vi "AlliGator Save All Decay Fit Parameter Maps to ASCII.vi"(8 "error in (no error)":errorcluster, 11 "Data Value Reference in":refnum<data-value>) -> (0 "error out":errorcluster, 3 "Data Value Reference out":refnum<data-value>)   [LabVIEW 2021, in "AlliGator Decay Fit Parameter Map.lvlib"]
doc: "Saves the Decay Fir Parameter Map 2D array to an ASCII file."
uses:
  AlliGator Decay Fit Parameter Map.lvlib
  AlliGator Internal Variables v2.ctl
  <vilib>/vision/Image Controls.llb/IMAQ Image.ctl
  AlliGator Gate Image Set.ctl
  AlliGator FLI Dataset Type.ctl
  AlliGator Data Series Type.ctl
  AlliGator Dataset Channel.ctl
  AlliGator Gate Arithmetic.ctl
  AlliGator Displayed Image.ctl
  Image/Named ROI Description.ctl
  AlliGator Decay Metadata v3.ctl
  AlliGator Decay Background Subtraction Info.ctl
  AlliGator Baseline Subtraction Method.ctl
  Graphs/XY Graph/XY Graph Plot Shift Parameters.ctl
  Graphs/XY Graph/XY Graph Plot Shift Method.ctl
  AlliGator Decay Extrapolation Parameters.ctl
  Phasor/Calibration Phasor (m, phi).ctl
  Phasor/Phasor Reference Series.ctl
  Phasor/Phasor Calibration Map v2.ctl
  Phasor/Phasor (g, s).ctl
  AlliGator Raw Phasor Plot Data v4.ctl
  Phasor/Phasor Standard Deviation Options.ctl
  AlliGator Phasor Multi-Harmonic Data.ctl
  Phasor/Phasor Harmonic Data.ctl
  AlliGator Decay Fit Options & Parameters v2.ctl
  Fits/IRF(X)PSED/Decay Fit Options v2.ctl
  Fits/Decay Convolution/Decay Model.ctl
  Fits/Residual Type.ctl
  Fits/IRF(X)PSED/Fit Weights Type.ctl
  Fits/Non-linear Fitting Method v2.ctl
  Fits/Fit Calculation Method.ctl
  Fits/Non-linear Fitting Algorithm.ctl
  AlliGator Decay Fit Parameter Constraints 2.ctl
  Fits/IRF(X)PSED/Decay Fit Parameters In List.ctl
  Fits/IRF(X)PSED/MLE Baseline Offset Type.ctl
  AlliGator Decay Preprocessing Parameters.ctl
  Fits/IRF(X)PSED/Decay Fit Parameters & Derived Quantities List.ctl
  AlliGator Parameter Maps Data.ctl
  AlliGator Variables List.ctl
  Variant/Variant to Data/Variant to U16.vi
  <vilib>/Utility/file.llb/Write Delimited Spreadsheet (DBL).vi
  AlliGator Files.lvlib
  Files/Files.lvlib
  Strings/Strings.lvlib
  GUI/GUI.lvlib
  Error/Error.lvlib
  Notebook/Notebook.lvlib
  Rich Text Box/Rich Text Box.lvlib
  AlliGator Globals, Variables & Constants.lvlib
  Variant/Variant to Data/Variant to Data.lvlib
  Phasor/Phasor.lvlib
  Image/Image.lvlib
  AlliGator Decay Preprocessing.lvlib
  Graphs/XY Graph/XY Graph Add-Ons.lvlib
  AlliGator Phasor Graph.lvlib
  AlliGator Phasor Plot.lvlib
  AlliGator Source Image.lvlib
  Fits/Fits.lvlib
  AlliGator Internal Variables.lvlib
  AlliGator Decay Fit.lvlib
  AlliGator Settings.lvlib
  AlliGator Dual-Channel Datasets.lvlib
panel:
  # "see the AlliGator License on the block diagram (Ctrl+E or Window:Show Block Diagram)"
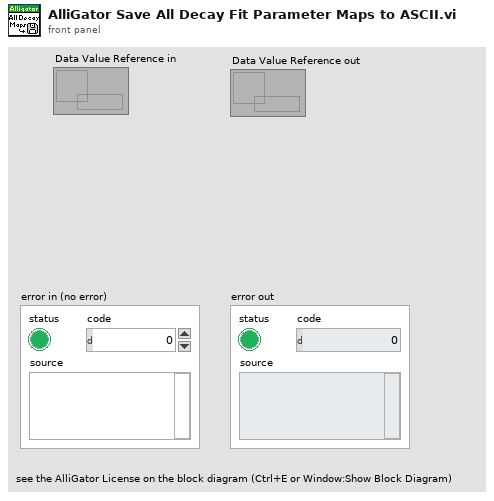
[diagram p1: front panel]
types:
  T1 = typedef "AlliGator Globals, Variables & Constants.lvlib/AlliGator Variables List.ctl" = enum16{"---- GUI ----", "GUI:Initialization Status", "GUI:State Indicators Refnum", "GUI:Original AlliGator Menu Items", "GUI:Current Action Loop State", "GUI:Script in progress", "GUI:Playback", "GUI:Loop Playback", "GUI:Search ROI Used", "GUI:Search ROI", "Decay Graph Max Legend Size", "Intensity Graph Max Legend Size", "Decay Statistics Graph Max Legend Size", "Phasor Graph Max Legend Size", "Phasor Ratio Graph Max Legend Size", "Lifetime Graph Max Legend Size", "---- Files ----", "Files:Export Dataset Frames as Individual Files", "Files:Show Batch Export Help Balloons", "Files:Frames in Dataset", "Files:ptu File Frame Start Indices", "Files:Current Frame in Dataset", "Files:Current Frame Timestamp", "Files:Dataset Loaded", "Files:Dataset Metadata", "Files:Dataset Channel", "Files:Dataset Data Description", "Files:Background Dataset Metadata", "Files:Background Dataset Channel", "Files:Background Dataset Data Description", "Files:Background File Subtraction", "Files:Background File Path", "Files:Background File Pile-up Correction", "Files:Background File Pixel Well Capacity", "Files:Background File Scaling Factor", "Files:Current Dataset Load Settings", "Files:Dataset Path", "Files:ICCD-specific Information", "Files:Macrotime Gate Separation", "------ Python Plugins ------", "Python Plugins:Information", "Python Plugins:Python Session", "Python Plugins:Valid Python Session?", "---- Source Image ----", "Source Image:ROIs", "Source Image:Current ROI", "Source Image:ROI Event Refnum", "X_Source Image Display Range", "X_Source Image Palette Information", "X_Type of Displayed Image", "X_Time Gate Slider", "Source Image:Palette List", "Source Image:Scale", "Source Image:ROI Overlay Color", "Source Image:Overlay to Erase", "Source Image:Is Displayed Image Accumulated", "Source Image:White Light Image Modified", "Source Image:Mask Image Modified", "---- Image Profile Window ----", "Image Profile:Window Event Refnum", "Image Profile:IntensityType", "Image Profile:Intensity Average Type", "Image Profile:Intensity-weighted SDV", "Image Profile:Box Profile Type", "Image Profile:Window Open", "Image Profile:Plotted Fit Parameter", "------ Phasor Graph -------", "Phasor Graph:Show Line", "---- Phasor Plot ---", "Phasor Plot:Parameters Changed", "Phasor Plot:FLI Dataset Modified since last Calculation", "Phasor Harmonics Data", "Selected Phasor Harmonics", "Phasor Harmonic Manager Event Refnum", "Phasor Plot:ROIs", "Phasor Plot:Current ROI", "Phasor Plot:ROI Event Refnum", "Phasor Plot:Image Reference Points", "Phasor Plot:Computed", "Phasor Plot:Palette Information", "Phasor Plot:Palette List", "Phasor Plot:Phasor Ratio Palette Information", "Phasor Plot:Phasor Ratio Palette List", "Phasor Plot:Image Scale", "Phasor Plot:Image Overlay to Erase", "Phasor Plot:Image Elements to Update", "Phasor Plot:Current Calculation Parameters", "Phasor Plot:Current Calibration Options", "Phasor Plot:Reset Cumulated Phasor Plot", "Phasor Plot:Reference 1", "Phasor Plot:Lifetime Reference 1", "Phasor Plot:Reference 1 Frequency", "Phasor Plot:Reference 2", "Phasor Plot:Lifetime Reference 2", "Phasor Plot:Reference 2 Frequency", "---- Decay Analysis ----", "Number of Selected Decays to Fit", "LS Fit Results", "LAR Fit Results", "BS Fit Results", "Last Decay Max - Min", "Best Fit Parameters", "Best Fit Parameter Names", "Actual Size X", "Actual Size Y", "Binning X", "Binning Y", "Actual # Gates", "Dataset Number", "Gates to...", "Gates Skipped", "Gates to keep", "Gate Step", "Gate Separation", "Reversed Gates", "Pile-up Correction", "Pixel Well Capacity", "Background Subtracted", "Background Subtraction Method", "Background Definition Range", "Background File (deprecated)", "Number of Dataset Accumulated", "Array of Accumulated Dataset Paths", "Do Averaged Datasets", "Destination File Path", "Process Plot Target", "Use 1/D as Phasor Frequency", "---- Decay Fit Parameter Map -----", "Decay Fit Parameter Map:Palette Information", "Decay Fit Parameter Map:Palette List", "------- Local Decay Window ---------", "Local Decay Graph Window:Event Refnum", "Local Decay Graph Window:Use normalized IRF for convolution", "----- Miscellaneous ----", "Misc:Skippable Dialog Windows Status"}
  T2 = typedef "IMAQ Image.ctl" = refnum<image>
  T3 = typedef "AlliGator Internal Variables.lvlib/AlliGator Internal Variables v2.ctl" = cluster{"Displayed Image":T2, "White Light Image":T2, "Mask Image":T2, "ROI Mask Image":T2, "Current Dataset Images 1":T4, "Background Dataset Images 1":T4, "Current Dataset Images 2":T4, "Background Dataset Images 2":T4, "Current Dataset Arithmetic Images":T4, "Accumulated Dataset Images 1":T4, "Accumulated Dataset Images 2":T4, "Accumulated Dataset Arithmetic Images":T4, "Phasor Plot Image":T2, "Decay Fit Parameter Map Image":T2, "Single Data Point Path":path, "White Light Image Path":path, "Mask Image Path":path, "Time-Series Folder":path, "[Time-Series Paths]":path[], "Current Dataset":i32, "Single Dataset Type":T5, "Current Folder":string, "AlliGator Data Series Type":T6, "# Datasets":i32, "Dual-Channel Dataset":bool, "Selected Channel Name":string, "Dataset Channel":T7, "Channel Arithmetic":T8, "Dual-Channel Background Dataset":bool, "Background Channel":T7, "Dual-Channel Accumulated Dataset":bool, "Start Time":dbl, "[Time-Series Timestamps]":dbl[], "[Intensity Corrections]":dbl[], "Time Series Script":bool, "Type of Displayed Image":T9, "Gate Image Slide":u16, "# Gates":i32, "ROIs":T10[], "ROI Decay":cluster{"t Array":dbl[], "I Array":dbl[]}, "Valid Decay":bool, "Decay  Metadata":T12, "Reference Decay Plot Name":string, "Reference Decay":cluster{"t Array":dbl[], "I Array":dbl[]}, "Decay Shift Plot":cluster{"Time Stamps":dbl[], "Decay Shifts":dbl[]}, "[Decays Max Values]":sgl[], "[Decays Min Values]":sgl[], "Calibration Phasor":T18, "Calibration Phasor Series":T19, "Phasor Calibration Map":T20, "Calibration Map MD5 Digest":string, "Last Raw Phasor":T21, "Last Calibrated Phasor":T21, "Last Calibrated Phasor SDV":T21, "Phasor Graph:Phasor Plot":cluster{"g Array":dbl[], "s Array":dbl[]}, "Phasor Graph:Phasor SDV Plot":cluster{"g Array":dbl[], "s Array":dbl[]}, "[Phasor Graph:Raw Phasor Plots]":T22[], "Phasor Plot locked to Ref 1":i32, "[Phasor Plot(s) locked to Ref 1]":i32[], "[Phasor Plot(s) locked to Ref 2]":i32[], "[Pixel Phasors]":T21[], "[[Sum Image]]":dbl[][], "[[CSG Phasors]]":csg[][], "[[Valid Pixel?]]":bool[][], "I/m/phi Dataset":cluster{"I/m/phi Dataset?":bool, "Base Frequency":dbl[unit], "Harmonic Orders":u8[]}, "Multi Phasor Plot Data":T24, "Decay Fit Options & Parameters":T26, "Fit Options: Decay Preprocessing Parameters":T37, "Fit Options: Reference Decay":cluster{"t Array":dbl[], "I Array":dbl[]}, "Is Full Image Parameters Map":bool, "Is Single-Pixels Parameters Map":bool, "NLSF Parameters Map X Resolution":i32, "NLSF Parameters Map Y Resolution":i32, "[Single Decay Fit Parameters]":dbl[], "Fit Model":T28, "[[Multiple Decays Fit Parameters]]":dbl[][], "[[Multiple Decays Fit Parameter SDVs]]":dbl[][], "[[IRFs]]":dbl[][], "IRF Array Time Axis":dbl[], "Decay Array Time Axis":dbl[], "[Decay Fit Parameter Names]":T38[], "[[Phasor Ratios]]":dbl[][], "[[Average Lifetimes]]":dbl[][], "Amplitude Weighted Average Lifetime":bool, "[Decay Sum]":dbl[], "Parameter Maps":T39[], "[[User-defined Quantities]]":dbl[][], "User-defined Quantity":string}
  T4 = typedef "AlliGator Internal Variables.lvlib/AlliGator Gate Image Set.ctl" = cluster{"SGL Image Max":T2, "SGL Image Sum":T2, "SGL Gate Images":T2[], "SGL Image Min":T2}
  T5 = typedef "AlliGator Files.lvlib/AlliGator FLI Dataset Type.ctl" = enum16{"HDF5 FLI Dataset", "Gate Image Folder", ".sdt FLI Dataset (Becker & Hickl)", ".ptu FLI Dataset (PicoQuant)", "SS1 FLI Dataset", "SS2 FLI Dataset", "I/m/phi Dataset", ".bin FLI Dataset (PicoQuant Binned)", ".bin FLI Dataset (Piccolo Binned)"}
  T6 = typedef "AlliGator Files.lvlib/AlliGator Data Series Type.ctl" = enum16{"Not a Supported Series", "Gate Images Folder Series", "SwissSPAD 2 Dataset Series", "B&H FLI Dataset Series", "PicoQuant PTU FLI Dataset Series", "PicoQuant BIN FLI Dataset Series", "Piccolo hist BIN FLI Dataset Series", "HDF5 FLI Dataset Series"}
  T7 = typedef "AlliGator Dual-Channel Datasets.lvlib/AlliGator Dataset Channel.ctl" = enum16{"G2", "INT"}
  T8 = typedef "AlliGator Settings.lvlib/AlliGator Gate Arithmetic.ctl" = enum16{"None", "INT-G2", "G2/INT*<INT>", "(1 - G2/INT)*<INT>"}
  T9 = typedef "AlliGator Source Image.lvlib/AlliGator Displayed Image.ctl" = enum16{"Single Gate", "Sum of All Gates", "Max of All Gates", "Min of All Gates", "-", "White Ligth Image", "Mask Image"}
  T10 = typedef "Image.lvlib/Named ROI Description.ctl" = cluster{"ROI Descriptor":T11, "ROI Name":string, "Overlay Color":u32}
  T11 = typedef "ROI Descriptor" = cluster{"Global Rectangle":i32[], "Contours":cluster{"ID":enum32{"External", "Internal"}, "Type":u32, "Coordinates":i32[]}[]}
  T12 = typedef "AlliGator Phasor Graph.lvlib/AlliGator Decay Metadata v3.ctl" = cluster{"ROI Descriptor":T11, "ROI Center":cluster{"X":i32, "Y":i32}, "Decay Background Subtraction Info":T13, "Decay Reverted":bool, "Decay Smoothened":bool, "Decay Straightened":bool, "Fitted Tau (Decay Straightening)":dbl, "Decay Shift Parameters":T15, "Decay Shifted":bool, "Decay Extrapolated":bool, "Decay Extrapolation Parameters":T17, "Decay Normalized":bool, "Fold Decay":bool, "# Folds":u32}
  T13 = typedef "AlliGator Decay Analysis.lvlib/AlliGator Decay Preprocessing.lvlib/AlliGator Decay Background Subtraction Info.ctl" = cluster{"Laser Period":dbl[unit], "Gate Duration":dbl[unit], "Baseline Subtraction Method":T14, "Background Definition Range":cluster{"Min Gate":dbl[unit], "Max Gate":dbl[unit]}, "Total Intensity w/o Bkgd Subtraction":dbl, "Bkgd-subtracted Intensity (exp)":dbl, "# Data Points":i32, "Background/Gate":dbl, "Fitted Lifetime":dbl[unit], "Bkgd-subtracted Intensity (theo)":dbl}
  T14 = typedef "AlliGator Decay Analysis.lvlib/AlliGator Decay Preprocessing.lvlib/AlliGator Baseline Subtraction Method.ctl" = enum16{"Mean", "Min", "Square Gated Single-Exponential", "File", "Constant"}
  T15 = typedef "XY Graph Add-Ons.lvlib/XY Graph Plot Shift Parameters.ctl" = cluster{"Type":T16, "Shift":dbl[unit], "Threshold":dbl, "Rotate":bool}
  T16 = typedef "XY Graph Add-Ons.lvlib/XY Graph Plot Shift Method.ctl" = enum16{"Default", "CFD", "Threshold", "Cross-Correlation"}
  T17 = typedef "AlliGator Decay Analysis.lvlib/AlliGator Decay Preprocessing.lvlib/AlliGator Decay Extrapolation Parameters.ctl" = cluster{"Additional Points":u32, "Head Fraction":dbl, "Fitted Tau":dbl, "Use Periodicity":bool, "Use Cursors":bool, "Tail Fraction":dbl}
  T18 = typedef "Phasor.lvlib/Calibration Phasor (m, phi).ctl" = cluster{"m":dbl, "phi":dbl, "Phasor Frequency":dbl[unit], "Reference Lifetime":dbl[unit]}
  T19 = typedef "Phasor.lvlib/Phasor Reference Series.ctl" = cluster{"m Array":dbl[], "phi Array":dbl[], "Phasor Frequency":dbl[unit], "Calibration Lifetime":dbl[unit]}
  T20 = typedef "Phasor.lvlib/Phasor Calibration Map v2.ctl" = cluster{"Phasor Frequency":dbl[unit], "Calibration Lifetime":dbl[unit], "ROI Centers":cluster{"X":i32, "Y":i32}[], "ROI Descriptors":T11[], "Map Resolution X":i32, "Map Resolution Y":i32, "z Array":cdb[]}
  T21 = typedef "Phasor.lvlib/Phasor (g, s).ctl" = cluster{"g":dbl, "s":dbl}
  T22 = typedef "AlliGator Phasor Graph.lvlib/AlliGator Raw Phasor Plot Data v4.ctl" = cluster{"Phasor Plot Name":string, "Raw Phasor Plot":T21[], "Phasor Frequency":dbl[unit], "[Decay Metadata]":T12[], "Raw Phasor Plot SDV":T21[], "Phasor SDV Options":T23, "[Calibration Phasor]":T18[]}
  T23 = typedef "Phasor.lvlib/Phasor Standard Deviation Options.ctl" = cluster{"Compute Estimated SDV":bool, "# Replicas":u32, "Use Estimated Average Phasor":bool}
  T24 = typedef "AlliGator Phasor Plot.lvlib/AlliGator Phasor Multi-Harmonic Data.ctl" = cluster{"Base Frequency":dbl[unit], "# Harmonics":u8, "Harmonic Orders":u8[], "Phasor Plot Settings Checksum":u64, "Phasor Harmonic Data Array":T25[]}
  T25 = typedef "Phasor.lvlib/Phasor Harmonic Data.ctl" = cluster{"Phasor Harmonic Name":string, "Phasor Plot Settings Checksum":u64, "Phasor Frequency":dbl[unit], "Base Frequency":dbl[unit], "Harmonic Order":u8, "Phasor Plot Parameters":string, "Phasor Array [[CSG]]":csg[][], "Dataset File Path":path}
  T26 = typedef "AlliGator Decay Fit Parameter Map.lvlib/AlliGator Decay Fit Options & Parameters v2.ctl" = cluster{"SYNC Period":dbl[unit], "Fit Options":T27, "Fit Parameter Constraints":T34[], "MLE Baseline Offset":dbl, "MLE Baseline Offset Type":T36}
  T27 = typedef "Fits.lvlib/Decay Fit Options v2.ctl" = cluster{"Show Fit Residuals":bool, "Fit Model":T28, "Residual Type":T29, "Max Decay Percentile":dbl, "Min Decay Percentile":dbl, "Show Full Decay":bool, "Weights":T30, "Fitting Method":T31, "Compute Parameter Uncertainties":bool, "Periodic Boundaries":bool, "Model Calculation":T32, "Period":dbl[unit], "Termination Criteria":cluster{"Max Iterations":i32, "Max Function Calls":i32, "Max Time":dbl[unit], "Function Tolerance":dbl, "Parameter Tolerance":dbl, "Gradient Tolerance":dbl, "Min Lambda":dbl, "Max Lambda":dbl, "Initial Tick Count":u32}, "Offset Resolution":dbl[unit], "Use Local IRF":bool, "Fitting Algorithm":T33}
  T28 = typedef "Fits.lvlib/Decay Model.ctl" = enum16{"1-Exponential", "2-Exponentials"}
  T29 = typedef "Fits.lvlib/Residual Type.ctl" = enum16{"Standard", "Normalized", "Reduced"}
  T30 = typedef "Fits.lvlib/Fit Weights Type.ctl" = enum16{"Unweighted", "1/Variance", "Best of All"}
  T31 = typedef "Fits.lvlib/Non-linear Fitting Method v2.ctl" = enum16{"Least Square", "Least Absolute Residual", "Bisquare", "MLE", "-", "Best of All"}
  T32 = typedef "Fits.lvlib/Fit Calculation Method.ctl" = enum16{"Simulation", "Convolution", "Integration"}
  T33 = typedef "Fits.lvlib/Non-linear Fitting Algorithm.ctl" = enum16{"Levenberg-Marquardt", "Trust-Region Dogleg"}
  T34 = typedef "AlliGator Decay Analysis.lvlib/AlliGator Decay Fit.lvlib/AlliGator Decay Fit Parameter Constraints 2.ctl" = cluster{"Fit Parameter":T35, "Min Value":dbl, "Max Value":dbl, "Global":bool, "Used":bool}
  T35 = typedef "Fits.lvlib/Decay Fit Parameters In List.ctl" = enum16{"Offset", "Baseline", "A_1", "tau_1", "A_2", "tau_2"}
  T36 = typedef "Fits.lvlib/MLE Baseline Offset Type.ctl" = enum32{"Absolute", "Percentage"}
  T37 = typedef "AlliGator Decay Analysis.lvlib/AlliGator Decay Preprocessing.lvlib/AlliGator Decay Preprocessing Parameters.ctl" = cluster{"Background Subtraction":bool, "Straighten Decay":bool, "Reverse Gates":bool, "1-Normalized Decay":bool, "Smoothen Decay":bool, "Smoothing Parameter":dbl, "Shift Decay":bool, "Decay Shift Parameters":T15, "Extrapolate Decay":bool, "Additional Points":u32, "Head Fraction":dbl, "Pixel-Normalize Decay":bool, "Use Periodicity":bool, "Use Cursors":bool, "Tail Fraction":dbl, "Use Decay Pre-Processing":bool, "Fold Decay":bool, "# Folds":u32, "[0-1]-Normalized Decay":bool}
  T38 = typedef "Fits.lvlib/Decay Fit Parameters & Derived Quantities List.ctl" = enum16{"Offset", "Baseline", "A_1", "tau_1", "A_2", "tau_2", "<tau>_a", "f1_a", "f2_a", "<tau>_i", "f1_i", "f2_i", "-", "R^2", "Chi^2"}
  T39 = typedef "AlliGator Parameter Maps Data.ctl" = cluster{"Map Set Name":string, "[Parameter Names]":string[], "[[Parameters]]":dbl[][], "[[Parameter SDVs]]":dbl[][], "Decay Array Time Axis":dbl[], "[[IRFs]]":dbl[][], "IRF Array Time Axis":dbl[]}
  T40 = typedef "Rich Text Box.lvlib/Text Formatting.ctl" = cluster{"Font":string, "Text Color":T41, "Text Background Color":T41, "Text Style":enum16{"Regular", "Bold", "Italic", "Underline", "Strikeout"}, "Font Size (Points)":dbl, "Text Alignment":i32}
  T41 = typedef "Rich Text Box.lvlib/Text Colors.ctl" = enum16{"Unchanged", "Black", "Blue", "Brown", "Gray", "Green", "Orange", "Pink", "Red", "White"}
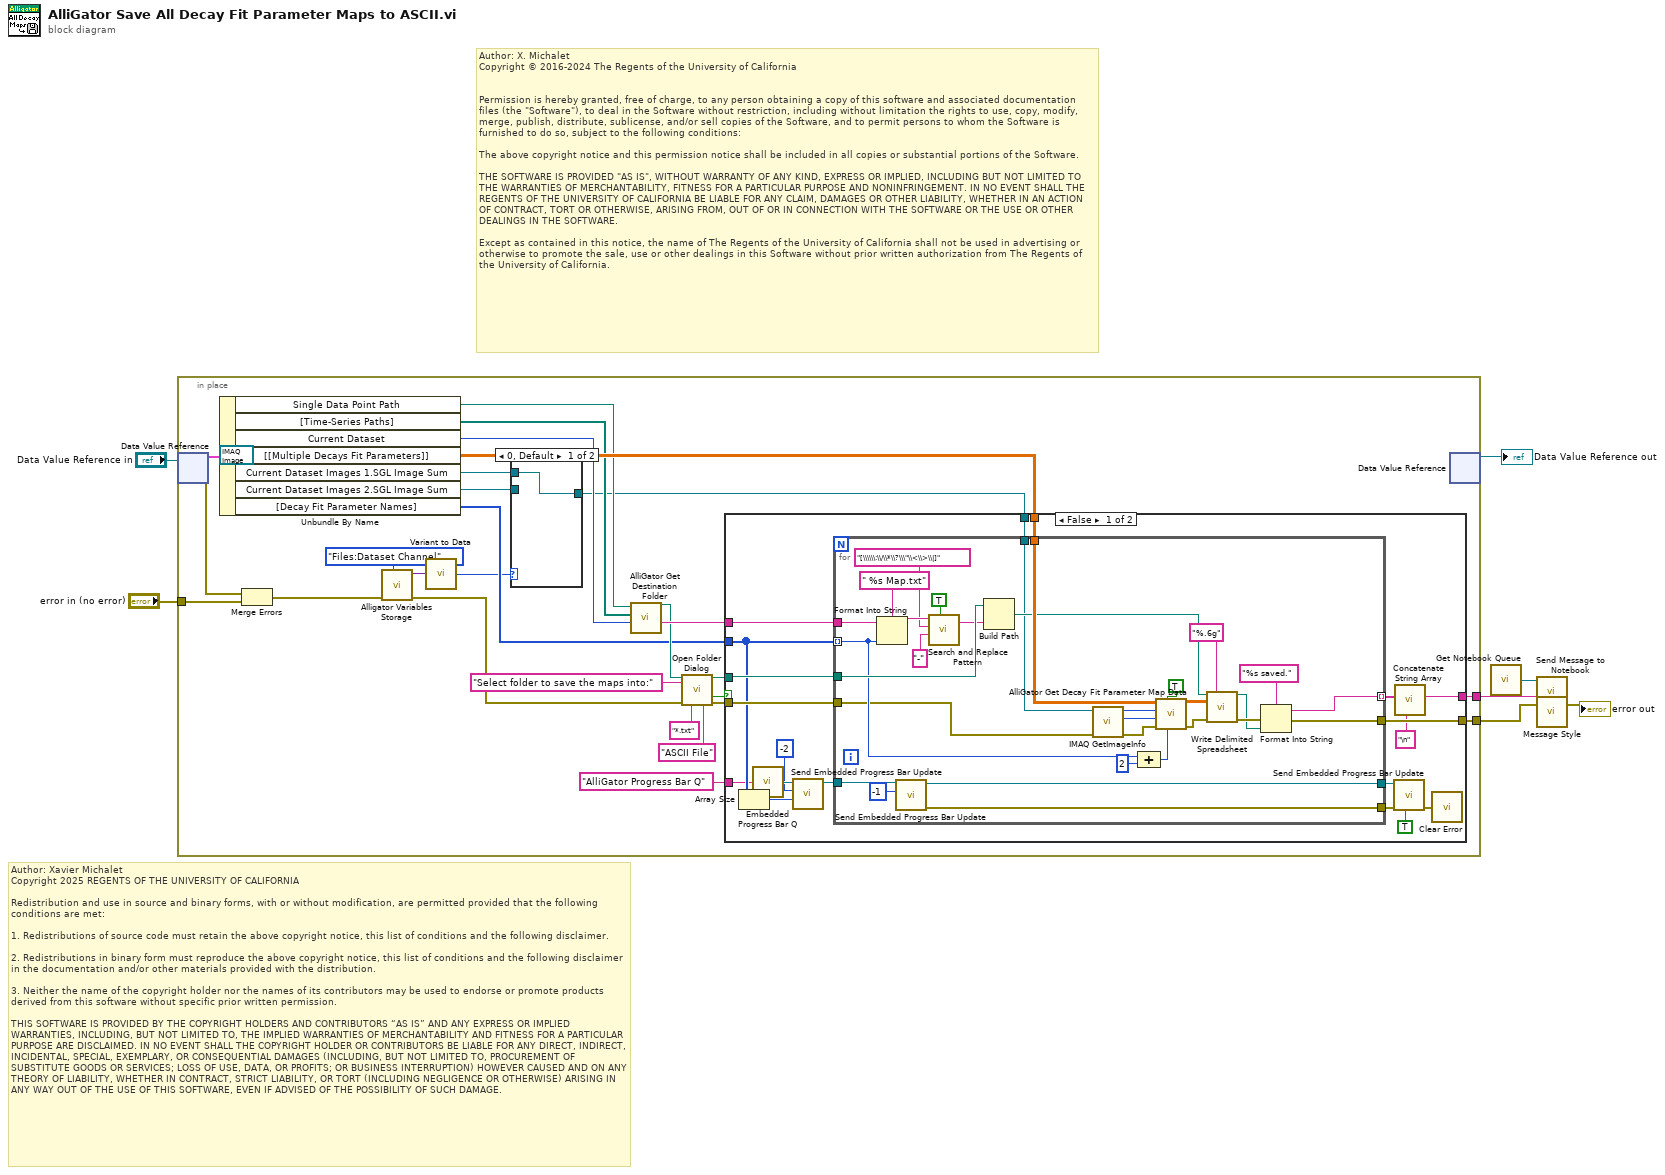
[diagram p0: block diagram]
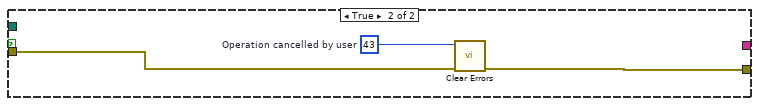
[diagram p2: hidden frame]
diagram:
  # "Author: Xavier Michalet\nCopyright 2025 REGENTS OF THE UNIVERSITY OF CALIFORNIA\n\nRedistribution and use in source and binary forms, with or without modification, are permitted provided that the following conditions are met:\n\n1. Redistributions of source code must retain the above copyright notice, this list of conditions and the following disclaimer.\n\n2. Redistributions in binary form must reproduce the above copyright notice, this list of conditions and the following disclaimer in the documentation and/or other materials provided with the distribution.\n\n3. Neither the name of the copyright holder nor the names of its contributors may be used to endorse or promote products derived from this software without specific prior written permission.\n\nTHIS SOFTWARE IS PROVIDED BY THE COPYRIGHT HOLDERS AND CONTRIBUTORS “AS IS” AND ANY EXPRESS OR IMPLIED WARRANTIES, INCLUDING, BUT NOT LIMITED TO, THE IMPLIED WARRANTIES OF MERCHANTABILITY AND FITNESS FOR A PARTICULAR PURPOSE ARE DISCLAIMED. IN NO EVENT SHALL THE COPYRIGHT HOLDER OR CONTRIBUTORS BE LIABLE FOR ANY DIRECT, INDIRECT, INCIDENTAL, SPECIAL, EXEMPLARY, OR CONSEQUENTIAL DAMAGES (INCLUDING, BUT NOT LIMITED TO, PROCUREMENT OF SUBSTITUTE GOODS OR SERVICES; LOSS OF USE, DATA, OR PROFITS; OR BUSINESS INTERRUPTION) HOWEVER CAUSED AND ON ANY THEORY OF LIABILITY, WHETHER IN CONTRACT, STRICT LIABILITY, OR TORT (INCLUDING NEGLIGENCE OR OTHERWISE) ARISING IN ANY WAY OUT OF THE USE OF THIS SOFTWARE, EVEN IF ADVISED OF THE POSSIBILITY OF SUCH DAMAGE."
  # "Author: X. Michalet\nCopyright © 2016-2024 The Regents of the University of California\n \n\nPermission is hereby granted, free of charge, to any person obtaining a copy of this software and associated documentation files (the \"Software\"), to deal in the Software without restriction, including without limitation the rights to use, copy, modify, merge, publish, distribute, sublicense, and/or sell copies of the Software, and to permit persons to whom the Software is furnished to do so, subject to the following conditions:\n\nThe above copyright notice and this permission notice shall be included in all copies or substantial portions of the Software.\n\nTHE SOFTWARE IS PROVIDED \"AS IS\", WITHOUT WARRANTY OF ANY KIND, EXPRESS OR IMPLIED, INCLUDING BUT NOT LIMITED TO THE WARRANTIES OF MERCHANTABILITY, FITNESS FOR A PARTICULAR PURPOSE AND NONINFRINGEMENT. IN NO EVENT SHALL THE REGENTS OF THE UNIVERSITY OF CALIFORNIA BE LIABLE FOR ANY CLAIM, DAMAGES OR OTHER LIABILITY, WHETHER IN AN ACTION OF CONTRACT, TORT OR OTHERWISE, ARISING FROM, OUT OF OR IN CONNECTION WITH THE SOFTWARE OR THE USE OR OTHER DEALINGS IN THE SOFTWARE.\n\nExcept as contained in this notice, the name of The Regents of the University of California shall not be used in advertising or otherwise to promote the sale, use or other dealings in this Software without prior written authorization from The Regents of the University of California."
  n1 = in-place {
    in-place-border: "error in (no error)" -> [w34]
    in-place-border: [w32] -> w2
    in-place-border: [w31] -> w3
    (unwired) T2 refnum ("Current Dataset Images.Image Sum")
    n2 = in-place-dvr #1("Data Value Reference in") -> (w35:T3, w33:errorcluster)
    n3 = Unbundle By Name(w35) -> ("Single Data Point Path"=w28:path, "[Time-Series Paths]"=w27:path[], "Current Dataset"=w26:i32, "[[Multiple Decays Fit Parameters]]"=w29:dbl[][], "Current Dataset Images 1.SGL Image Sum"=w9:T2, "Current Dataset Images 2.SGL Image Sum"=w16:T2, "[Decay Fit Parameter Names]"=w18:T38[])
    n4 = Merge Errors(w33, w34) -> (w12:errorcluster)
    n5 = call "Alligator Variables Storage.vi"("AlliGator Variable"=AlliGator_Variables_List."Files:Dataset Channel" ("Alligator Variable"), "Error In"=w12) -> ("Error Out"=w11:errorcluster, "Data out"=w13:variant)  [unwired: 7 in, 1 out]
    n6 = call-poly "Variant to Data.vi"("Variant"=w13) -> ("U16 Value"=w10:u16)  [unwired: 8 in]
    n7 = case shown="0, Default" w10 {
      tunnel: [w89 w90] -> w15
      tunnel: w16 -> [_ w90]
      tunnel: w9 -> [w89 _]
      frame 0, Default {
      }
      frame 1 {
      }
    }
    n8 = call "AlliGator Get Destination Folder.vi"("Current Data Set (-1: single)"=w26, "Time-Series Paths"=w27, "Single Data Point Path"=w28) -> ("Data Point Name"=w30:string, "Destination Folder path"=w22:path)  [unwired: 6 in, 1 out]
    n9 = call "Open Folder Dialog.vi"("start path"=w22, "prompt"="Select folder to save the maps into:", "error in"=w11, "pattern (all files)"="*.txt", "pattern label"="ASCII File") -> ("selected path"=w20:path, "cancelled"=w21:bool, "error out"=w19:errorcluster)  [unwired: 7 in, 1 out]
    n10 = case shown="False" w21 {
      tunnel: w30 -> [w54 _]
      tunnel: w29 -> [w53 _]
      tunnel: w15 -> [w52 _]
      tunnel: [w51 w87] -> w32
      tunnel: [w47 _] -> w31
      tunnel: w20 -> [w50 _]
      tunnel: w19 -> [w49 w88]
      tunnel: w18 -> [w45 _]
      tunnel: "AlliGator Progress Bar Q" ("Progress Bar Queue Name") -> [w44 _]
      frame False {
        n11 = Array Size(array=w45) -> (size(s)=w37:i32)
        n12 = call "Embedded Progress Bar Q.vi"("Progress Bar Queue Name"=w44) -> ("Progress Bar Queue"=w39:refnum<queue>)  [unwired: 6 in]
        n13 = call "Send Embedded Progress Bar Update.vi"("Max Iterations N"=w37, "Current Iteration i (i or -1: standard or || iteration; 0 or -2: first standard or || iteration)"=-2 ("Current Iteration i (i or -1: standard or || iteration; 0 or -2: first standard or || iteration)"), "Progress Bar Queue in"=w39) -> ("Progress Bar Queue out"=w38:refnum<queue>)  [unwired: 7 in, 1 out]
        n14 = for {
          tunnel: w54 -> [w85]
          tunnel: w53 -> [w83]
          tunnel: w52 -> [w81]
          tunnel: [w80] -> w51
          tunnel: [w79] -> w48 mode=indexing
          tunnel: w50 -> [w78]
          tunnel: w45 -> [w66] mode=indexing
          tunnel: w49 -> [w65]
          tunnel: w38 -> [w63]
          tunnel: [w62] -> w43
          tunnel: [w61] -> w42
          n15 = Format Into String(format string=" %s Map.txt", initial string=w85, w66) -> (resulting string=w58:string)  [unwired: 1 in, 1 out]
          n16 = call "Send Embedded Progress Bar Update.vi"("Current Iteration i (i or -1: standard or || iteration; 0 or -2: first standard or || iteration)"=-1 ("Current Iteration i (i or -1: standard or || iteration; 0 or -2: first standard or || iteration)"), "Progress Bar Queue in"=w63) -> ("Error Out"=w61:errorcluster, "Progress Bar Queue out"=w62:refnum<queue>)  [unwired: 8 in]
          n17 = call <vilib>:"Search and Replace Pattern.vi"("string"=w58, "regular expression (\"\")"="[\\\\\\:\\/\\*\\?\\\"\\<\\>\\|]" ("format string"), "replace string (\"\")"="-" ("replace string (\"\")"), "replace all? (F)"=TRUE) -> ("result string"=w59:string)  [unwired: 1 in, 1 out]
          n18 = Build Path(base path=w78, name or relative path=w59) -> (appended path=w82:path)
          n19 = call "IMAQ GetImageInfo"("error in (no error)"=w65, "Image"=w81) -> ("error out"=w73:errorcluster, "Y Resolution"=w74:i32, "X Resolution"=w75:i32)  [unwired: 2 in, 5 out]
          n20 = Compound Arithmetic op=unknown(w66, 2 ("value")) -> (w76:i32)
          n21 = call "AlliGator Get Decay Fit Parameter Map Data.vi"("Map index"=w76, "Compute Decay Fit Parameter Map"=TRUE, "Error In"=w73, "Y Resolution"=w74, "X Resolution"=w75, "Multiple Decays Fit Parameters"=w83) -> ("Error Out"=w64:errorcluster, "Map Data (V x H)"=w71:dbl[][])  [unwired: 3 in, 1 out]
          n22 = call-poly <vilib>:"Write Delimited Spreadsheet.vi"("file path (dialog if empty)"=w82, "format (%.3f)"="%.6g", "2D data"=w71, "error in (no error)"=w64) -> ("new file path (Not A Path if cancelled)"=w67:path, "error out"=w69:errorcluster)  [unwired: 10 in]
          n23 = Format Into String(format string="%s saved.", error in=w69, w67) -> (resulting string=w79:string, error out=w80:errorcluster)  [unwired: 1 in]
        }
        n24 = call "Send Embedded Progress Bar Update.vi"("Stop Progress Bar (F)"=TRUE, "Error In"=w42, "Progress Bar Queue in"=w43) -> ("Error Out"=w40:errorcluster)  [unwired: 7 in, 1 out]
        n25 = call "Concatenate String Array.vi"("Separator (TAB)"="\n", "String Array"=w48) -> ("Formatted String"=w47:string)  [unwired: 9 in]
        n26 = call "Clear Error.vi"("Error In"=w40) -> ()  [unwired: 8 in, 1 out]
      }
      frame True {
        w86 = 43  # Operation cancelled by user
        n27 = call <vilib>:"Clear Errors.vi"("error in (no error)"=w88, "specific error code to clear (0: all)"=w86) -> ("error out"=w87:errorcluster)  [unwired: 4 in, 1 out]
      }
    }
    n28 = in-place-dvr #1() -> (→"Data Value Reference out":refnum<data-value>)  [unwired: 1 in, 1 out]
  }
  n29 = call "Get Notebook Queue.vi"() -> ("Notebook Queue"=w4:refnum<queue>)  [unwired: 9 in]
  n30 = call "Message Style.vi"() -> ("Message Formatting"=w5:T40)
  n31 = call "Send Message to Notebook.vi"("Text Formatting"=w5, "Error In"=w2, "Message"=w3, "Notebook Queue"=w4) -> ("Error Out"=→"error out":errorcluster)  [unwired: 4 in, 1 out]
